vi "[Dynamic Call] Selection.vi"(7 "VI Refnum":refnum<vi>, 9 "Start Coords":T1, 10 "Config":T2={"Selection"={"caption"="", "Validaty Threshold"=0, "Color"=6618880, "Start Coords"={"Horizontal"=0, "Vertical"=0}}, "Cursor"={"Name"="", "Position"={"X"=0.0, "Y"=0.0}}}, 11 "GrphChrt Refnum":refnum<vi>) -> ()   [LabVIEW 2019]
uses:
  [Selection] Config.ctl
  <vilib>/Utility/miscctls.llb/LVPoint32TypeDef.ctl
  <vilib>/Utility/miscctls.llb/LVPointDoubleTypeDef.ctl
  Graph Tools.lvlib
panel:
  out "error out":errorcluster
  in  "error in (no error)":errorcluster
  out "reference out":refnum<vi>
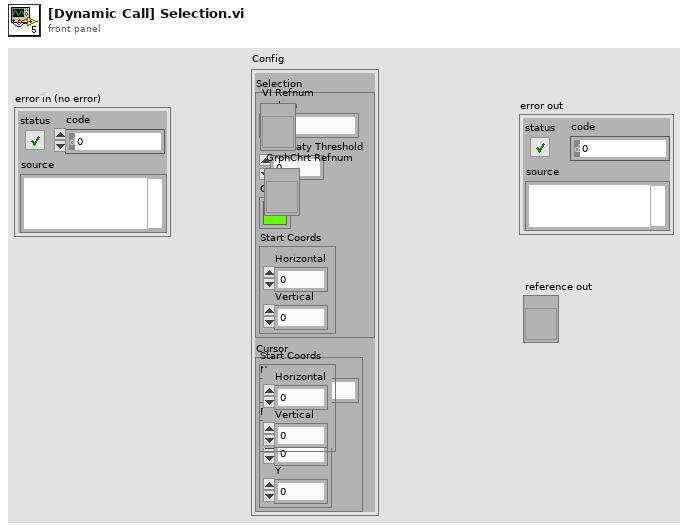
[diagram p1: front panel]
types:
  T1 = typedef "LVPoint32TypeDef.ctl" = cluster{"Horizontal":i32, "Vertical":i32}
  T2 = typedef "Graph Tools.lvlib/[Selection] Config.ctl" = cluster{"Selection":cluster{"caption":string, "Validaty Threshold":i32, "Color":u32, "Start Coords":T1}, "Cursor":cluster{"Name":string, "Position":T3}}
  T3 = typedef "LVPointDoubleTypeDef.ctl" = cluster{"X":dbl, "Y":dbl}
  T4 = cluster{"Control Name":string, "Value":variant}[]
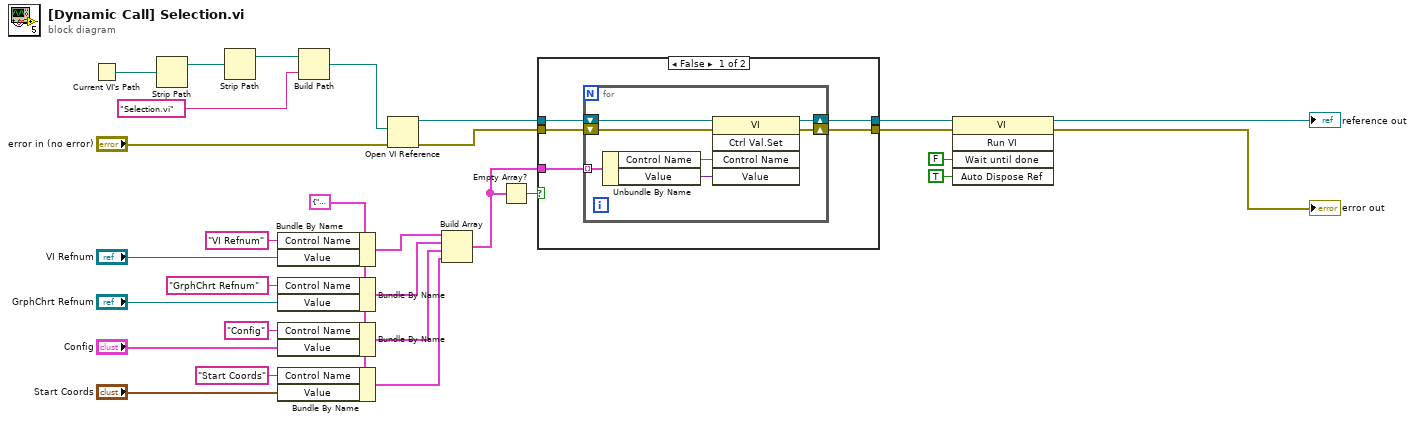
[diagram p0: block diagram]
diagram:
  w6 = cluster{"Control Name":string, "Value":variant} {"Control Name"="", "Value"=variant} ("Control Values")
  n1 = Current VI's Path() -> (path=w19:path)
  n2 = Strip Path(path=w19) -> (stripped path=w10:path)  [unwired: 1 out]
  n3 = Strip Path(path=w10) -> (stripped path=w9:path)  [unwired: 1 out]
  n4 = Bundle By Name(cluster=w6, "Control Name"="VI Refnum", "Value"="VI Refnum") -> (w3:cluster{"Control Name":string, "Value":variant})
  n5 = Bundle By Name(cluster=w6, "Control Name"="GrphChrt Refnum", "Value"="GrphChrt Refnum") -> (w4:cluster{"Control Name":string, "Value":variant})
  n6 = Bundle By Name(cluster=w6, "Control Name"="Config", "Value"="Config") -> (w5:cluster{"Control Name":string, "Value":variant})
  n7 = Bundle By Name(cluster=w6, "Control Name"="Start Coords", "Value"="Start Coords") -> (w13:cluster{"Control Name":string, "Value":variant})
  n8 = Build Path(base path=w9, name or relative path="Selection.vi") -> (appended path=w17:path)
  n9 = Open VI Reference(vi path=w17, error in (no error)="error in (no error)") -> (vi reference=w21:refnum<vi>, error out=w20:errorcluster)  [unwired: 4 in]
  n10 = Build Array(w3, w4, w5, w13) -> (w12:T4)
  n11 = Empty Array?(array=w12) -> (empty?=w24:bool)
  n12 = case shown="False" w24 {
    tunnel: w21 -> [w34 w43]
    tunnel: [w33 w43] -> w23
    tunnel: w20 -> [w32 w42]
    tunnel: [w30 w42] -> w22
    tunnel: w12 -> [w31 _]
    frame False {
      n13 = for {
        shift-right: [w40] -> w33
        shift-left: w34 -> [w41]
        shift-right: [w38] -> w30
        shift-left: w32 -> [w39]
        tunnel: w31 -> [w37] mode=indexing
        n14 = Unbundle By Name(w37) -> ("Control Name"=w36:string, "Value"=w35:variant)
        n15 = invoke class="VI" method="Ctrl Val.Set"(reference=w41, error in=w39, "Control Name"=w36, "Value"=w35) -> (reference out=w40:refnum<vi>, error out=w38:errorcluster)  [unwired: 1 in, 3 out]
      }
    }
    frame True {
    }
  }
  n16 = invoke class="VI" method="Run VI"(reference=w23, error in=w22, "Wait until done"=FALSE ("Wait Until Done"), "Auto Dispose Ref"=TRUE ("Auto Dispose Reference")) -> (reference out=→"reference out":refnum<vi>, error out=→"error out":errorcluster)  [unwired: 1 in, 3 out]
